vi "Get Files and Folders.vi"(0 "File Directory":path, 11 "error in (no error)":errorcluster) -> (4 "Files and Folders":path[](array[path]), 6 "Files and Folder Names":string[](array[string]), 15 "error out":errorcluster)   [LabVIEW 2021, in "Packager Helpers.lvlib"]
uses:
  Packager Helpers.lvlib
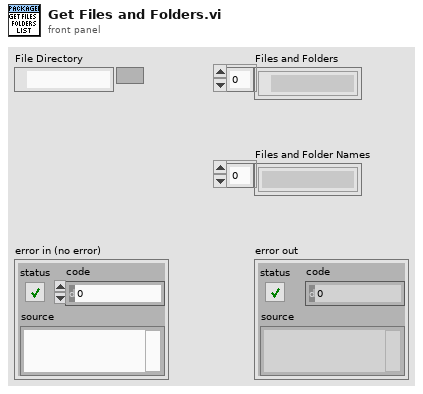
[diagram p1: front panel]
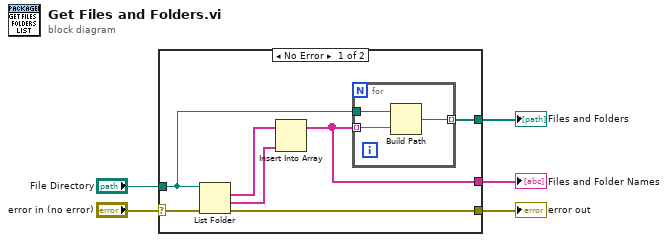
[diagram p0: block diagram]
diagram:
  n1 = case shown="No Error" "error in (no error)" {
    selector: "error in (no error)" -> [w8 w16]
    tunnel: [w9 _] -> w5
    tunnel: [w7 w16] -> w4
    tunnel: [w10 _] -> w3
    tunnel: "File Directory" -> [w6 _]
    frame No Error {
      n2 = List Folder(path=w6, error in=w8) -> (filenames=w12:string[], folder names=w11:string[], error out=w7:errorcluster)  [unwired: 2 in, 1 out]
      n3 = Insert Into Array(array=w12, new element=w11) -> (w9:string[])  [unwired: 1 in]
      n4 = for {
        tunnel: w6 -> [w15]
        tunnel: w9 -> [w14] mode=indexing
        tunnel: [w13] -> w10 mode=indexing
        n5 = Build Path(base path=w15, name or relative path=w14) -> (appended path=w13:path)
      }
    }
    frame Error {
    }
  }
  "Files and Folders" <- w3
  "error out" <- w4
  "Files and Folder Names" <- w5
